vi "APDM Get GPD Opals.vi"(0 "APDM Context":T1={"APDM Context ID"=0, "Gyro Mode"="", "Log Data"=FALSE, "Log File"=refnum, "Gyro Record Log"=refnum, "Gyro CMD Log"=refnum, "L Opal SN"=0, "R Opal SN"=0, "Access Point ID"=0, "Left Gyro Sim Data"=path "C:/Users/jfalesi/Desktop/CP FES Walking Code/Original/Ahad Vi/CP Code/Offline data/TD_7_Raw_R.txt", "Right Gyro Sim Data"=path "C:/Users/jfalesi/Desktop/CP FES Walking Code/Original/Ahad Vi/CP Code/Offline data/TD_7_Raw_R.txt", "Sampling Rate"=0.0, "Gyro Sim Time Array"=[], "Missed Gyro Count"=0.0}, 1 "error in (no error)":errorcluster) -> (2 "APDM Context":T1={"APDM Context ID"=0, "Gyro Mode"="", "Log Data"=FALSE, "Log File"=refnum, "Gyro Record Log"=refnum, "Gyro CMD Log"=refnum, "L Opal SN"=0, "R Opal SN"=0, "Access Point ID"=0, "Left Gyro Sim Data"=path "C:/Users/jfalesi/Desktop/CP FES Walking Code/Original/Ahad Vi/CP Code/Offline data/TD_7_Raw_R.txt", "Right Gyro Sim Data"=path "C:/Users/jfalesi/Desktop/CP FES Walking Code/Original/Ahad Vi/CP Code/Offline data/TD_7_Raw_R.txt", "Sampling Rate"=0.0, "Gyro Sim Time Array"=[], "Missed Gyro Count"=0.0}, 3 "Opal SNs":u32[](array[numeric])=[1510, 1801], 4 "error out":errorcluster)   [LabVIEW 2019]
uses:
  Controls/APDM Context Cluster.ctl
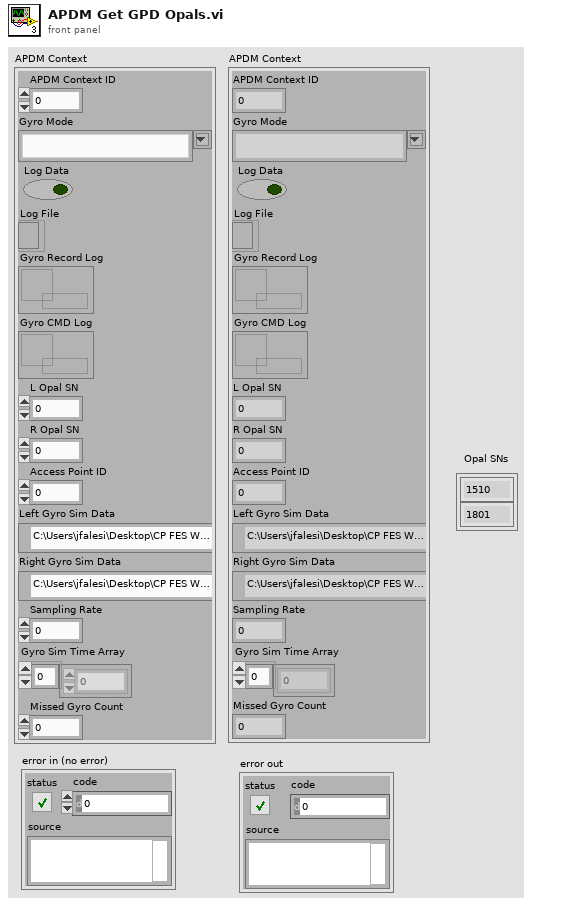
[diagram p1: front panel]
types:
  T1 = typedef "APDM Context Cluster.ctl" = cluster{"APDM Context ID":u32, "Gyro Mode":string, "Log Data":bool, "Log File":refnum<file>, "Gyro Record Log":refnum<queue>, "Gyro CMD Log":refnum<queue>, "L Opal SN":u32, "R Opal SN":u32, "Access Point ID":u32, "Left Gyro Sim Data":path, "Right Gyro Sim Data":path, "Sampling Rate":dbl, "Gyro Sim Time Array":dbl[], "Missed Gyro Count":dbl}
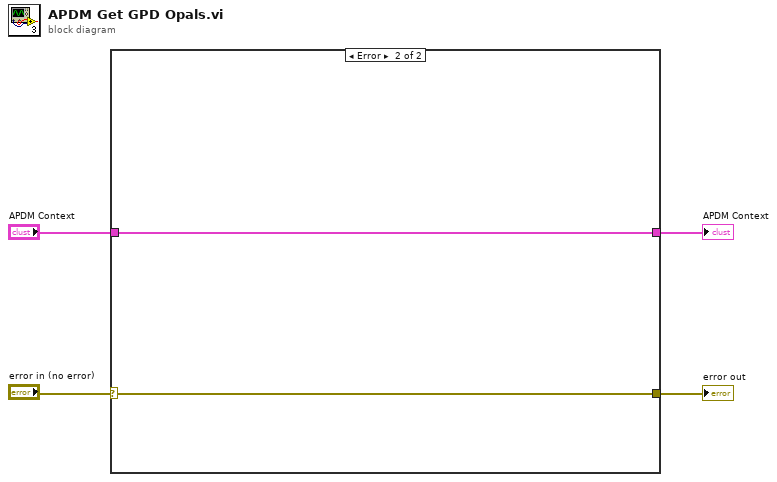
[diagram p0: block diagram]
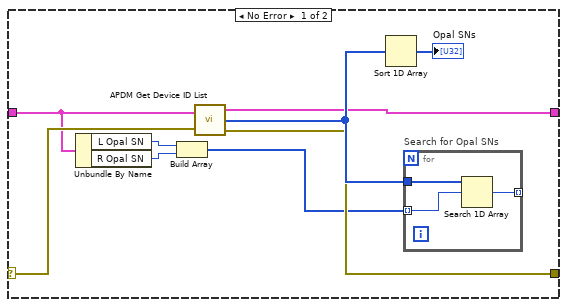
[diagram p2: hidden frame]
diagram:
  n1 = case shown="Error" "error in (no error)" {
    selector: "error in (no error)" -> [w7 w18]
    tunnel: [w11 w18] -> w4
    tunnel: "APDM Context" -> [w6 w17]
    tunnel: [w5 w17] -> w1
    frame No Error {
      n2 = Unbundle By Name(w6) -> ("L Opal SN"=w10:u32, "R Opal SN"=w9:u32)
      n3 = Build Array(w10, w9) -> (w8:u32[])
      n4 = call "APDM Get Device ID List.vi"("APDM Context"=w6, "error in (no error)"=w7) -> ("APDM Context"=w5:T1, "Device List"=w12:u32[], "error out"=w11:errorcluster)
      n5 = Sort 1D Array(array=w12) -> (sorted array=→"Opal SNs":u32[])
      n6 = for "Search for Opal SNs" {
        tunnel: w12 -> [w16]
        tunnel: [w15] -> _ mode=indexing
        tunnel: w8 -> [w14] mode=indexing
        n7 = Search 1D Array(1D array=w16, element=w14) -> (index of element=w15:i32)  [unwired: 1 in]
      }
    }
    frame Error {
    }
  }
  "error out" <- w4
  "APDM Context" <- w1
